vi "PS35_PhasePwmFreq.vi"(0 "Axis number":i32=1 min=1 max=3, 1 "Control unit ID":i32=1 min=1 max=10, 2 "Value-In":enum16{"20000", "80000"}(ring), 3 "error in (no error)":errorcluster, 5 "function":bool) -> (7 "Value-Out":i32, 9 "error out":errorcluster)   [LabVIEW 2020]
doc: "PS35_PhasePwmFreq.vi, created: 04.03.2009 alex; last change: 22.10.2019 alex;\n\n<B>FUNCTIONS:</B> \n\n<B>Read:</B> FALSE: read PWM frequency of the power amplifier \nfor an axis (values in Hz). \n<B>Write:</B> TRUE: set PWM frequency of the power amplifier \nfor an axis (values in Hz).\n----------------------------------------------------------------------------------------\n<B>INPUT:</B>\n[TF] <B>function:</B> function selector. (Read, Write)\n[I32] <B>Control unit ID:</B> control unit index. (Default=1, Range=1...10)\n[I32] <B>Axis number:</B> axis number. (Default=1, Range=1...3)\n[Enum] <B>Value-In:</B> PWM frequency (20000 or 80000 Hz). \n(only for Write: Default=0 - 20000 Hz, Range=0...1)\n[CLU] <B>error in</B>\n----------------------------------------------------------------------------------------\n<B>OUTPUT:</B>\n[I32] <B>Value-Out:</B> PWM frequency. \n(for Write: Value-Out=Value-In)\n[CLU] <B>error out</B>\n----------------------------------------------------------------------------------------\n<B>SUB-VIs:</B>\nPS35_GetReadError.vi\n----------------------------------------------------------------------------------------\n<B>EXT-Calls:</B>\nps35.dll (V2.01)\n----------------------------------------------------------------------------------------"
uses:
  ps35.dll
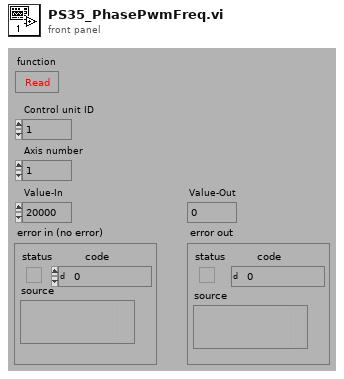
[diagram p1: front panel]
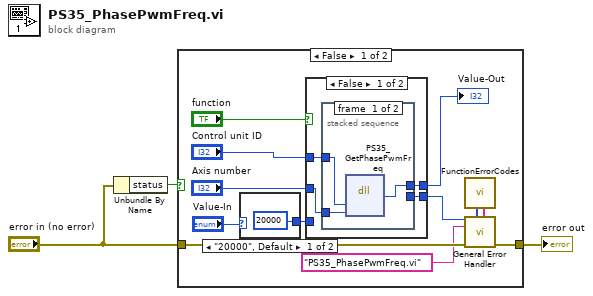
[diagram p0: block diagram]
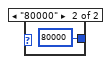
[diagram p2: hidden frame]
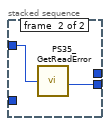
[diagram p3: hidden frame]
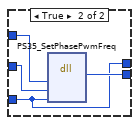
[diagram p4: hidden frame]
diagram:
  n1 = Unbundle By Name("error in (no error)") -> ("status"=w1:bool)
  n2 = case shown="False" w1 {
    tunnel: "error in (no error)" -> [w15 w31]
    tunnel: [w14 w31] -> w3
    frame False {
      n3 = case shown="\"20000\", Default" "Value-In" {
        tunnel: [20000 80000] -> w7
        frame "20000", Default {
        }
        frame "80000" {
        }
      }
      n4 = case shown="False" "function" {
        tunnel: "Control unit ID" -> [w20 w29]
        tunnel: [w21 w30] -> w11
        tunnel: w7 -> [_ w27]
        tunnel: [w19 w27] -> w10
        tunnel: "Axis number" -> [w18 w28]
        frame False {
          n5 = stacked-sequence {
            tunnel: [_ w26] -> w21
            tunnel: w20 -> [w24 w25]
            tunnel: [w23 _] -> w19
            tunnel: w18 -> [w22 _]
            frame #0 {
              n6 = dll-call lib="C:/GEECS/Developers Version/source/Device Drivers/OwiSoft/OWISoftOEM/ps35/labview/lv82/ps35.dll" fn="PS35_GetPhasePwmFreq" label="PS35_\nGetPhase\nPwmFreq"("Index"=w24, "AxisNr"=w22) -> ("Rückgabetyp"=w23:i32)  [unwired: 5 in, 2 out]
            }
            frame #1 {
              n7 = call "PS35_GetReadError.vi"("Control unit ID"=w25) -> ("Read error"=w26:i32)
            }
          }
        }
        frame True {
          n8 = dll-call lib="C:/GEECS/Developers Version/source/Device Drivers/OwiSoft/OWISoftOEM/ps35/labview/lv82/ps35.dll" fn="PS35_SetPhasePwmFreq" label="PS35_\nSetPhase\nPwmFreq"("Index"=w29, "AxisNr"=w28, "Value"=w27) -> ("Rückgabetyp"=w30:i32)  [unwired: 6 in, 2 out]
        }
      }
      "Value-Out" <- w10
      n9 = call "FunctionErrorCodes.vi"() -> ("[user-defined codes]"=w5:i32[], "[user-defined descriptions]"=w4:string[])  [unwired: 8 in]
      n10 = call <vilib>:"General Error Handler.vi"("[error code] (0)"=w11, "[user-defined codes]"=w5, "[user-defined descriptions]"=w4, "[error source] (\" \")"="PS35_PhasePwmFreq.vi" ("[error source] (\" \")"), "error in (no error)"=w15) -> ("error out"=w14:errorcluster)  [unwired: 6 in, 4 out]
    }
    frame True {
    }
  }
  "error out" <- w3
